vi "Set Temp Setpoint Data--Accessor.vi"(8 "error in (no error)":errorcluster, 10 "Temp Setpoint Data":T1, 11 "Simulated Thermal Process Controller in":refnum<class "Simulated Thermal Process Controller.lvclass">) -> (0 "error out":errorcluster, 3 "Simulated Thermal Process Controller out":refnum<class "Simulated Thermal Process Controller.lvclass">)   [LabVIEW 2024, in "Simulated Thermal Process Controller.lvclass"]
uses:
  Simulated Thermal Process Controller.lvclass
  Process Controller/Controls/Temp Data--Cluster.ctl
  Process Controller/Controls/Temperature Units--Enum.ctl
  Simulated Thermal Process Controller.lvclass/Simulated Thermal Process Controller.ctl
  Process Controller/_Thermal Process Controller.lvclass
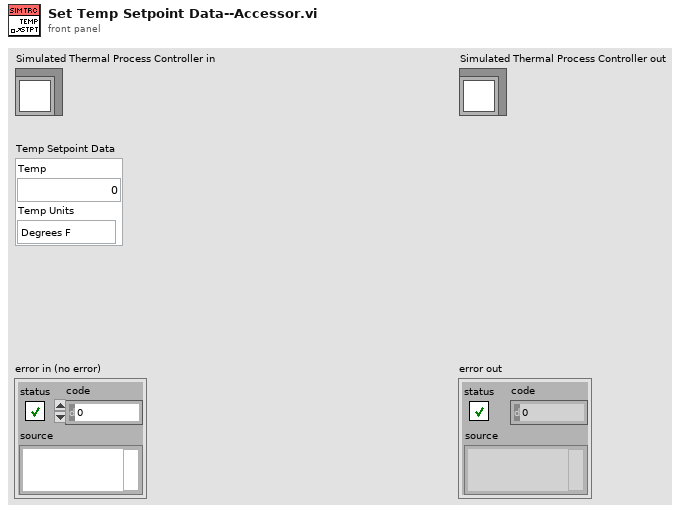
[diagram p1: front panel]
types:
  T1 = typedef "_Thermal Process Controller.lvclass/Temp Data--Cluster.ctl" = cluster{"Temp":dbl, "Temp Units":T2}
  T2 = typedef "_Thermal Process Controller.lvclass/Temperature Units--Enum.ctl" = enum16{"Degrees F", "Degrees C", "Degrees K"}
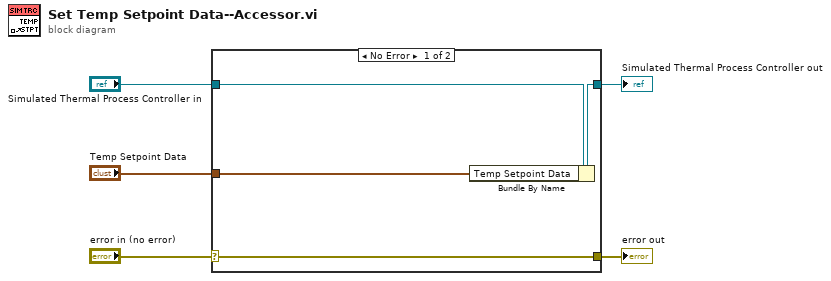
[diagram p0: block diagram]
diagram:
  n1 = case shown="No Error" "error in (no error)" {
    selector: "error in (no error)" -> [w9 w10]
    tunnel: [w9 w10] -> w4
    tunnel: [w7 w11] -> w2
    tunnel: "Simulated Thermal Process Controller in" -> [w8 w11]
    tunnel: "Temp Setpoint Data" -> [w6 _]
    frame No Error {
      n2 = Bundle By Name(cluster=w8, "Temp Setpoint Data"=w6) -> (w7:refnum<class "Simulated Thermal Process Controller.lvclass">)
    }
    frame Error {
    }
  }
  "error out" <- w4
  "Simulated Thermal Process Controller out" <- w2
